vi "CmdCluster2DesiredRow.vi"(11 "DesiredParameters":T1) -> (3 "DesiredStatRow":string[](array[string]))   [LabVIEW 2013]
uses:
  TypeDef/Command Cluster.ctl
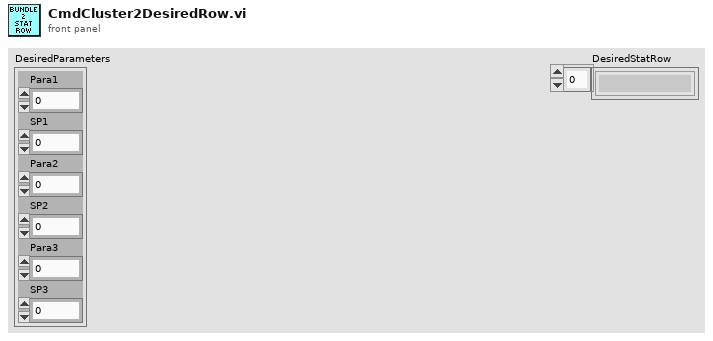
[diagram p1: front panel]
types:
  T1 = typedef "Command Cluster.ctl" = cluster{"Para1":i32, "SP1":dbl, "Para2":i32, "SP2":dbl, "Para3":i32, "SP3":dbl}
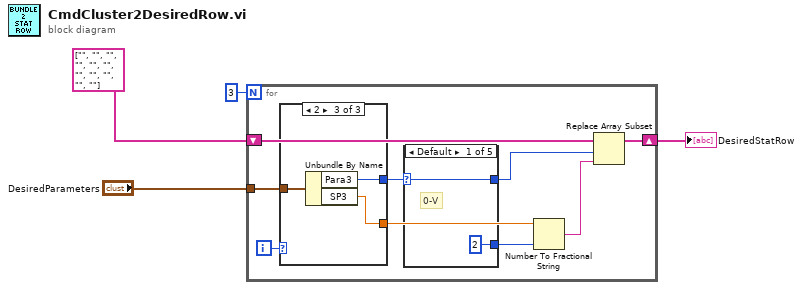
[diagram p0: block diagram]
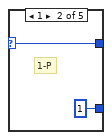
[diagram p2: hidden frame]
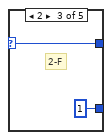
[diagram p3: hidden frame]
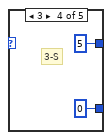
[diagram p4: hidden frame]
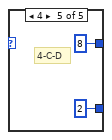
[diagram p5: hidden frame]
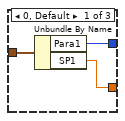
[diagram p6: hidden frame]
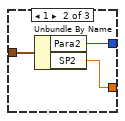
[diagram p7: hidden frame]
diagram:
  n1 = for {
    N: 3 -> [_]
    tunnel: "DesiredParameters" -> [w12]
    shift-right: [w10] -> w1
    shift-left: string[] ["", "", "", "", "", "", "", "", "", "", ""] -> [w11]
    i -> [w13]
    n2 = case shown="2" w13 {
      tunnel: w12 -> [w26 w29 w32]
      tunnel: [w25 w28 w31] -> w7
      tunnel: [w24 w27 w30] -> w9
      frame 0, Default {
        n3 = Unbundle By Name(w26) -> ("Para1"=w24:i32, "SP1"=w25:dbl)
      }
      frame 1 {
        n4 = Unbundle By Name(w29) -> ("Para2"=w27:i32, "SP2"=w28:dbl)
      }
      frame 2 {
        n5 = Unbundle By Name(w32) -> ("Para3"=w30:i32, "SP3"=w31:dbl)
      }
    }
    n6 = case shown="Default" w9 {
      selector: w9 -> [w15 w17 w19 _ _]
      tunnel: [w15 w17 w19 5 ("Para1") 8 ("Para1")] -> w8
      tunnel: [2 1 1 0 2] -> w5
      frame Default {
        # "0-V"
      }
      frame 1 {
        # "1-P"
      }
      frame 2 {
        # "2-F"
      }
      frame 3 {
        # "3-S"
      }
      frame 4 {
        # "4-C-D"
      }
    }
    n7 = Number To Fractional String(number=w7, precision (6)=w5) -> (F-format string=w6:string)  [unwired: 2 in]
    n8 = Replace Array Subset(array=w11, new element=w6, index=w8) -> (w10:string[])
  }
  "DesiredStatRow" <- w1
